vi "heatwarning.vi"() -> ()   [LabVIEW 2017]
panel:
  out "Weather Out":T1
  in  "Weather In":T1
  in  "error in (no error)":errorcluster
  out "error out":errorcluster
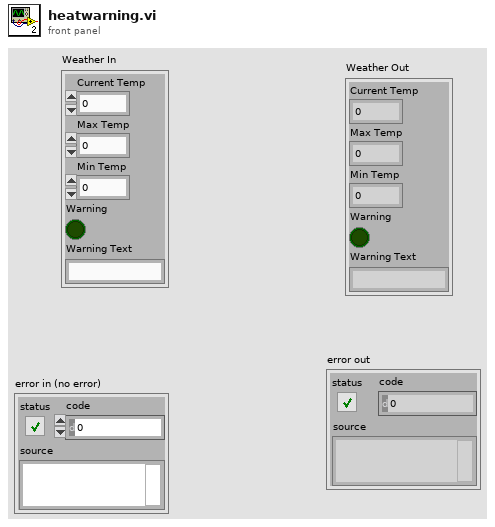
[diagram p1: front panel]
types:
  T1 = cluster{"Current Temp":dbl, "Max Temp":dbl, "Min Temp":dbl, "Warning":bool, "Warning Text":string}
  T2 = cluster{"Current Temp":dbl, "Max Temp":dbl, "Min Temp":dbl, bool, string}
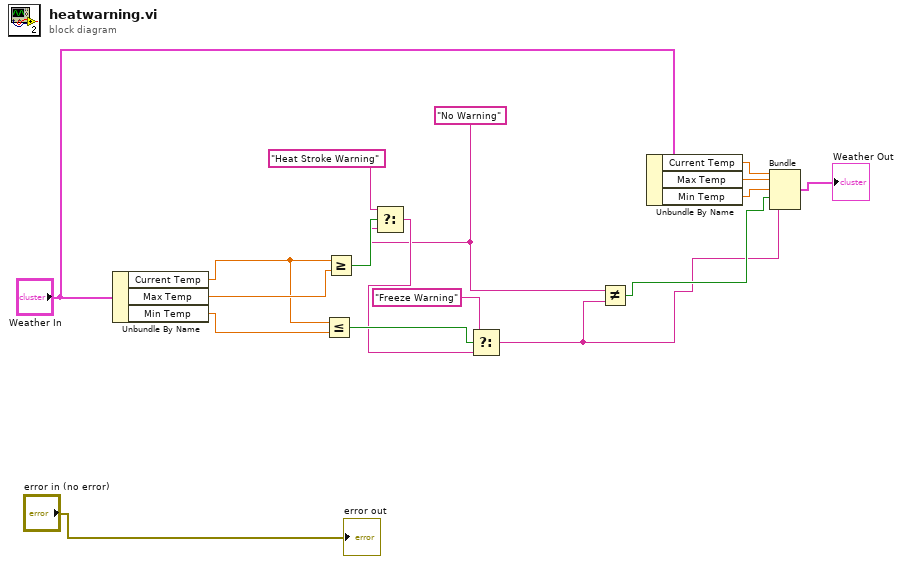
[diagram p0: block diagram]
diagram:
  w9 = "No Warning"
  n1 = Unbundle By Name("Weather In") -> ("Current Temp"=w16:dbl, "Max Temp"=w17:dbl, "Min Temp"=w15:dbl)
  n2 = Less Or Equal?(x=w16, y=w15) -> (x <= y?=w14:bool)
  n3 = Greater Or Equal?(x=w16, y=w17) -> (x >= y?=w12:bool)
  n4 = Select(t="Heat Stroke Warning", s=w12, f=w9) -> (s? t:f=w11:string)
  n5 = Select(t="Freeze Warning", s=w14, f=w11) -> (s? t:f=w2:string)
  n6 = Not Equal?(x=w9, y=w2) -> (x != y?=w3:bool)
  n7 = Unbundle By Name("Weather In") -> ("Current Temp"=w6:dbl, "Max Temp"=w5:dbl, "Min Temp"=w4:dbl)
  n8 = Bundle("Current Temp"=w6, "Max Temp"=w5, "Min Temp"=w4, w3, w2) -> (→"Weather Out":T2)  [unwired: 1 in]
  "error out" <- "error in (no error)"
